vi "removeSpace.vi"(8 "error in":errorcluster, 11 "input":string) -> (0 "error out":errorcluster, 3 "output":string)   [LabVIEW 2019]
doc: "Remove space in the name of a file."
uses:
  <vilib>/regexp/Match Regular Expression.xnode
  <vilib>/JDP Science/JDP Science Common Utilities/JDP Utility.lvlib
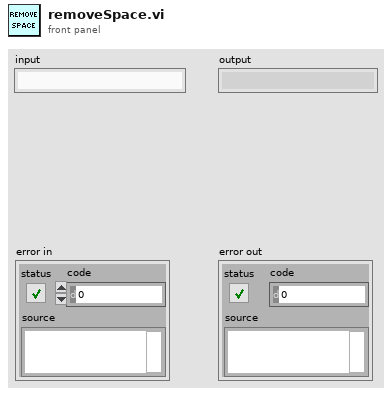
[diagram p1: front panel]
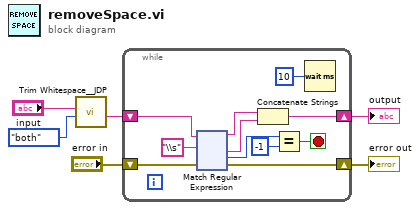
[diagram p0: block diagram]
diagram:
  n1 = call <vilib>:"Trim Whitespace__JDP.vi"("Remove (leading and trailing)"=enum16{"leading", "trailing", "both"}."both", "String in"="input") -> ("String out"=w1:string)  [unwired: 5 in]
  n2 = while {
    shift-right: [w16] -> w4
    shift-left: "error in" -> [w17]
    shift-right: [w9] -> w2
    shift-left: w1 -> [w8]
    stop <- w12 stop-if-true
    n3 = xnode "Match Regular Expression"("input string"=w8, "regular expression"="\\s", "error in"=w17) -> ("before match"=w11:string, "after match"=w10:string, "offset past match"=w14:i32, "error out"=w16:errorcluster)  [unwired: 3 in, 1 out]
    n4 = Concatenate Strings(w11, w10) -> (w9:string)
    n5 = Equal?(x=w14, y=-1) -> (x = y?=w12:bool)
    n6 = Wait (ms)(milliseconds to wait=u32 10) -> ()  [unwired: 1 out]
  }
  "error out" <- w4
  "output" <- w2
